vi "VirtualBench_Current_Measurement.vi"(8 "Error In":errorcluster, 9 "Acquisition Time (s)":dbl=10.0, 10 "Measure":i32(ring)=2 caption="Function (no change)" items=["DC Volts", "AC Volts", "DC Current", "AC Current", "Resistance", "Diode"], 11 "VB Device Name":tag="VirtualBench" caption="Device Name") -> (0 "Error Out":errorcluster, 3 "Average Value":dbl format="%#_6f")   [LabVIEW 2016]
uses:
  <vilib>/Platform/TimedLoop/XDataNode/timing_clust.ctl
  <vilib>/Platform/TimedLoop/XDataNode/nitl_modes.ctl
  <vilib>/Platform/TimedLoop/XDataNode/wakeup.ctl
  <vilib>/Analysis/baseanly.llb/Mean (DBL).vi
  <vilib>/VirtualBench/_DMM Configure Measurement0.vi
  <vilib>/platform/TimedLoop/XDataNode/XDataNode.xnode
  <vilib>/VirtualBench/VirtualBench.lvlib
  <vilib>/Platform/TimedLoop/XDataNode/XDNodeRunTimeDep.lvlib
  <vilib>/Analysis/NI_AALBase.lvlib
panel:
  out "Minimum Value":dbl format="%#_6f"
  out "Maximum Value":dbl format="%#_6f"
  out "Measured values":dbl[](array[numeric]) format="%#_6f"
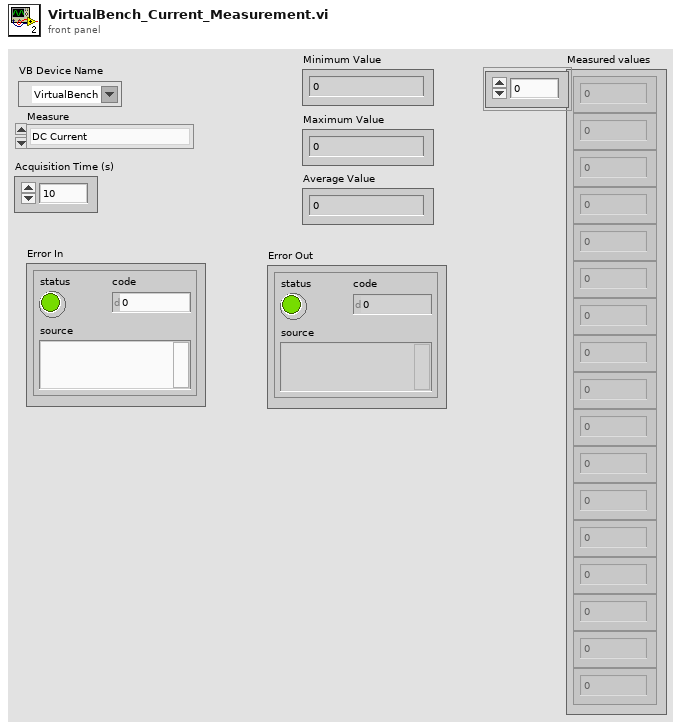
[diagram p1: front panel]
types:
  T1 = typedef "XDNodeRunTimeDep.lvlib/timing_clust.ctl" = cluster{"Expected End [f-1]":u64, "Actual End [f-1]":u64, "Finished Late? [f-1]":bool, "Expected End [i-1]":u64, "Actual End [i-1]":u64, "Finished Late? [i-1]":bool, "Expected Start [i]":u64, "Actual Start [i]":u64, "Expected Start [f]":u64, "Actual Start [f]":u64, "Source Name":string, "Structure Name":string, "Period":i64, "Deadline":i64, "Offset":i64, "Start":i64, "Priority":i32, "Timeout":i32, "Mode":T2, "Wakeup Reason":T3, "Error":errorcluster, "Source Type":string, "Secondary Source Type":string, "Global End Time":u64, "Global Start Time":u64, "Frame Duration":u64, "Iteration Duration":u64, "Assigned CPU":i32, "I/O Scan Engine Mode":u32}
  T2 = typedef "XDNodeRunTimeDep.lvlib/nitl_modes.ctl" = enum32{"No Change", "Process missed periods, maintain original phase", "Discard missed periods, maintain original phase", "Process missed periods, ignore original phase", "Discard missed periods, ignore original phase"}
  T3 = typedef "XDNodeRunTimeDep.lvlib/wakeup.ctl" = enum32{"Normal", "Aborted", "Asynchronous wakeup", "Timing source error", "Timed loop error", "Timeout"}
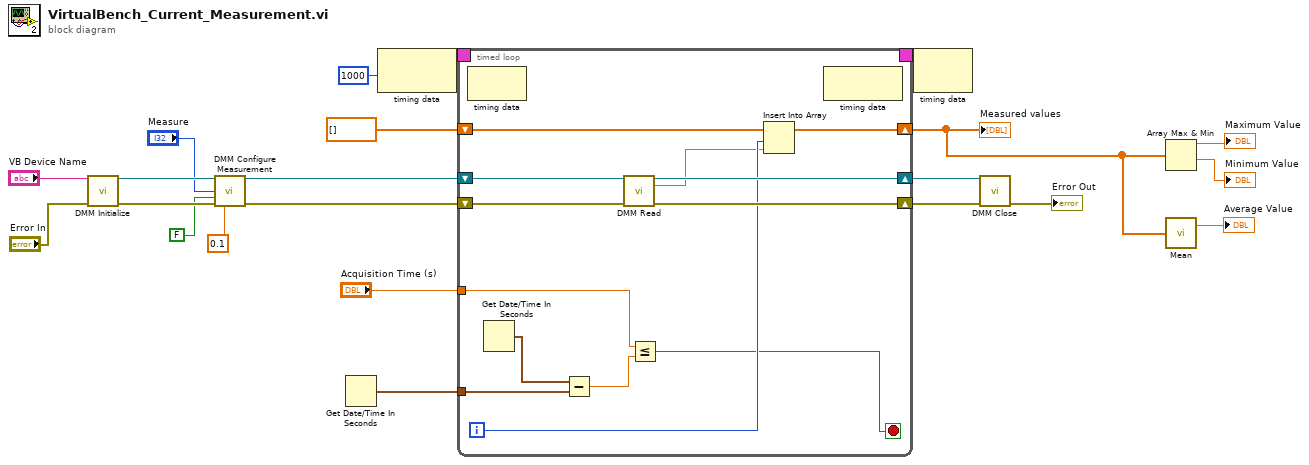
[diagram p0: block diagram]
diagram:
  n1 = call <vilib>:"DMM Initialize.vi"("Device Name"="VB Device Name", "Error In"="Error In") -> ("Instrument Handle Out"=w21:refnum<k21>, "Error Out"=w20:errorcluster)  [unwired: 12 in]
  n2 = call-poly <vilib>:"DMM Configure Measurement.vi"("Instrument Handle In"=w21, "Function"="Measure", "Auto Range"=FALSE, "Error In"=w20, "Manual Range"=0.1) -> ("Instrument Handle Out"=w19:refnum<k21>, "Error Out"=w18:errorcluster)  [unwired: 9 in]
  n3 = Get Date/Time In Seconds() -> (seconds since 1Jan1904=w8:timestamp)
  n4 = node-c288(i64 1000 ("Period")) -> (w11:T1)
  n5 = timed-loop {
    timing: w11 -> [_]
    timing-out: [_] -> w10
    shift-right: [w33] -> w17
    shift-left: w19 -> [w35]
    shift-right: [w32] -> w16
    shift-left: w18 -> [w34]
    shift-right: [w28] -> w5
    shift-left: dbl[] [] -> [w29]
    tunnel: w8 -> [w26]
    tunnel: "Acquisition Time (s)" -> [w25]
    i -> [w31]
    stop <- w23 stop-if-true
    n6 = node-c288() -> ()  [unwired: 1 in, 1 out]
    n7 = Get Date/Time In Seconds() -> (seconds since 1Jan1904=w27:timestamp)
    n8 = Subtract(x=w27, y=w26) -> (x-y=w24:dbl)
    n9 = call <vilib>:"DMM Read.vi"("Instrument Handle In"=w35, "Error In"=w34) -> ("Instrument Handle Out"=w33:refnum<k21>, "Measurement"=w30:dbl, "Error Out"=w32:errorcluster)  [unwired: 11 in]
    n10 = Less Or Equal?(x=w25, y=w24) -> (x <= y?=w23:bool)
    n11 = Insert Into Array(array=w29, index=w31, new element=w30) -> (w28:dbl[])
    n12 = node-c288() -> ()  [unwired: 1 in, 1 out]
  }
  "Measured values" <- w5
  n13 = node-c288(w10) -> ()  [unwired: 1 out]
  n14 = call <vilib>:"DMM Close.vi"("Instrument Handle In"=w17, "Error In"=w16) -> ("Error Out"=→"Error Out":errorcluster)  [unwired: 13 in]
  n15 = Array Max & Min(array=w5) -> (max value=→"Maximum Value":dbl, min value=→"Minimum Value":dbl)  [unwired: 2 out]
  n16 = call-poly <vilib>:"Mean.vi"("X"=w5) -> ("mean"=→"Average Value":dbl)  [unwired: 1 out]
